vi "mitsu.vi"() -> ()   [LabVIEW 2020]
panel:
  out "error out":errorcluster
  out "data out":u16
  in  "192.168.3.39_test":u16
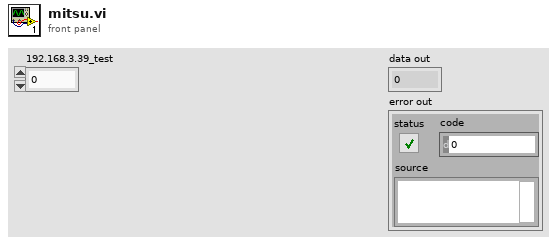
[diagram p1: front panel]
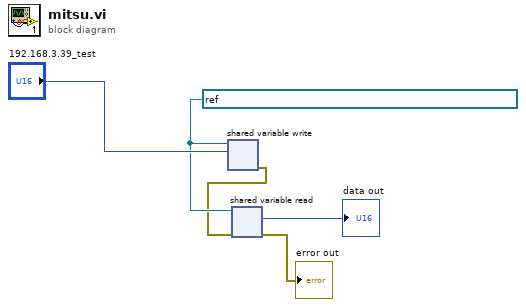
[diagram p0: block diagram]
diagram:
  w4 = refnum<k21> "ni.var.psp://localhost/TestOPC/OPC/HAVC/22/D409_0" ("shared variable refnum in")
  n1 = shared-variable-write(w4, "192.168.3.39_test") -> (w3:errorcluster)  [unwired: 1 in, 1 out]
  n2 = shared-variable-read(w4, w3) -> (→"error out":errorcluster, →"data out":u16)  [unwired: 1 out]
